vi "Call acquisition simulators.vi"() -> ()   [LabVIEW 2017]
uses:
  Rendezvous global.vi
panel:
  out "End":bool
  out "Calling acq. devs.":bool
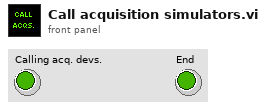
[diagram p1: front panel]
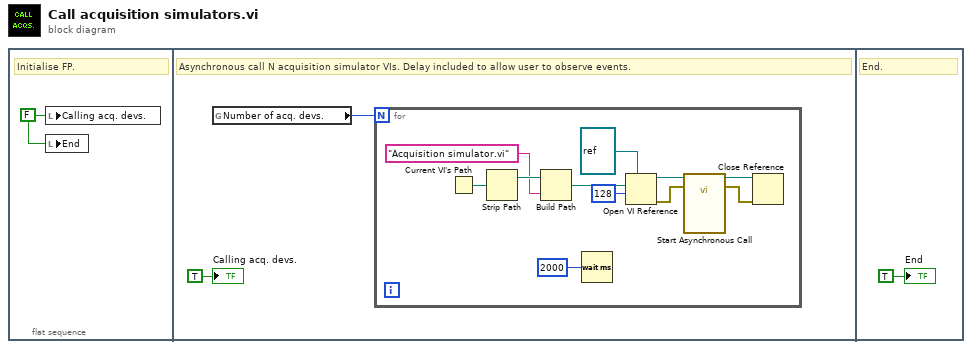
[diagram p0: block diagram]
diagram:
  n1 = flat-sequence {
    frame #0 {
      w1 = FALSE ("Calling 1")
      # "Initialise FP."
      n2 = local write "Calling acq. devs."(w1) -> ()
      n3 = local write "End"(w1) -> ()
    }
    frame #1 {
      # "Asynchronous call N acquisition simulator VIs. Delay included to allow user to observe events."
      n4 = global read "Rendezvous global.vi" "Number of acq. devs."() -> (w2:i32)
      n5 = for {
        N: w2 -> [_]
        n6 = Current VI's Path() -> (path=w11:path)
        n7 = Strip Path(path=w11) -> (stripped path=w10:path)  [unwired: 1 out]
        n8 = Build Path(base path=w10, name or relative path="Acquisition simulator.vi") -> (appended path=w8:path)
        n9 = Wait (ms)(milliseconds to wait=u32 2000) -> ()  [unwired: 1 out]
        n10 = Open VI Reference(type specifier VI Refnum (for type only)=refnum<vi> refnum, vi path=w8, options=128) -> (vi reference=w7:refnum<vi>, error out=w5:errorcluster)  [unwired: 3 in]
        n11 = call-by-ref "Start Asynchronous Call"(reference=w7, error in=w5) -> (reference out=w6:refnum<vi>, error out=w4:errorcluster)  [unwired: 1 in]
        n12 = Close Reference(reference=w6, error in (no error)=w4) -> ()  [unwired: 1 out]
      }
      "Calling acq. devs." <- TRUE ("Calling 1")
    }
    frame #2 {
      # "End."
      "End" <- TRUE ("Calling 1")
    }
  }
